vi "Web API Query.vi"(8 "error in (no error)":errorcluster, 11 "url":string="https://geocoding-api.open-meteo.com/v1/search?name=Nordheim&countryCode=DE&language=de&count=20") -> (0 "error out":errorcluster, 3 "API Response":string)   [LabVIEW 2025, in "UI Launcher.lvlib"]
uses:
  UI Launcher/UI Launcher.lvlib
  <vilib>/httpClient/LabVIEWHTTPClient.lvlib
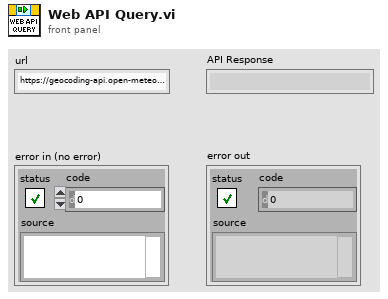
[diagram p1: front panel]
types:
  T1 = typedef "LabVIEWHTTPClient.lvlib/ClientHandle.ctl" = refnum<k1>
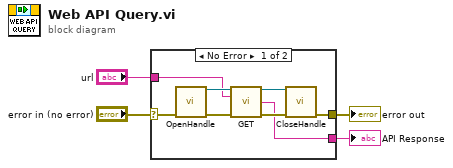
[diagram p0: block diagram]
diagram:
  n1 = case shown="No Error" "error in (no error)" {
    selector: "error in (no error)" -> [w6 w13]
    tunnel: "url" -> [w9 _]
    tunnel: [w7 _] -> w3
    tunnel: [w5 w13] -> w1
    frame No Error {
      n2 = call <vilib>:"OpenHandle.vi"("error in (no error)"=w6) -> ("client handle out"=w12:T1, "error out"=w10:errorcluster)  [unwired: 13 in]
      n3 = call <vilib>:"GET.vi"("client handle"=w12, "url"=w9, "error in (no error)"=w10) -> ("client handle out"=w11:T1, "body"=w7:string, "error out"=w8:errorcluster)  [unwired: 9 in, 1 out]
      n4 = call <vilib>:"CloseHandle.vi"("client handle"=w11, "error in (no error)"=w8) -> ("error out"=w5:errorcluster)  [unwired: 13 in]
    }
    frame Error {
    }
  }
  "API Response" <- w3
  "error out" <- w1
